vi "writeToXML.vi"(8 "error in (no error)":errorcluster, 10 "classLabel":string, 11 "SetEngineerAccessMode in":refnum<class "SetEngineerAccessMode.lvclass">) -> (0 "error out":errorcluster, 2 "XML out":string, 3 "SetEngineerAccessMode out":refnum<class "SetEngineerAccessMode.lvclass">)   [LabVIEW 2022 SP3, in "TCSDataDefinitions.lvlib" / "TCSCommand.lvlib" / "SetAccessMode.lvlib" / "SetEngineerAccessMode.lvclass"]
uses:
  SetEngineerAccessMode.lvclass
  SetEngineerAccessMode.lvclass/SetEngineerAccessMode.ctl
  SetAccessMode/SetAccessMode.lvclass
  <userlib>/Common/XML/XMLGenerator/XMLGenerator.lvclass
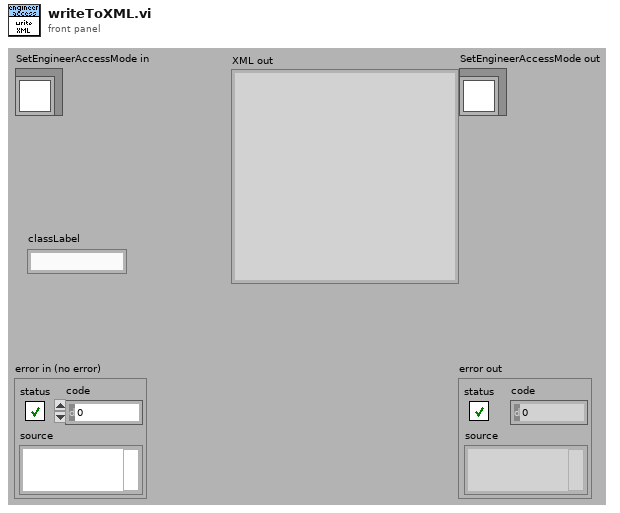
[diagram p1: front panel]
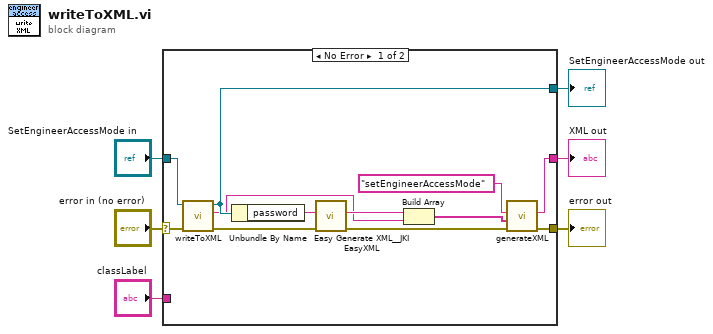
[diagram p0: block diagram]
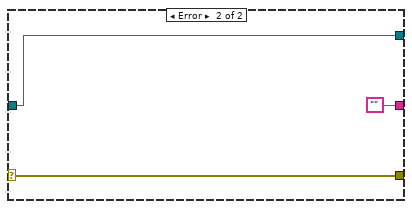
[diagram p2: hidden frame]
diagram:
  n1 = case shown="No Error" "error in (no error)" {
    selector: "error in (no error)" -> [w9 w21]
    tunnel: [w8 w21] -> w5
    tunnel: [w17 w20] -> w3
    tunnel: "SetEngineerAccessMode in" -> [w18 w20]
    tunnel: [w7 ""] -> w2
    tunnel: "classLabel" -> [_ _]
    frame No Error {
      n2 = call-parent "writeToXML.vi"("error in (no error)"=w9, "SetAccessMode in"=w18) -> ("error out"=w11:errorcluster, "XML out"=w14:string, "SetAccessMode out"=w17:refnum<class "SetEngineerAccessMode.lvclass">)  [unwired: 7 in]
      n3 = Unbundle By Name(w17) -> ("password"=w16:string)
      n4 = call <vilib>:"Easy Generate XML__JKI EasyXML.vi"("error in (no error)"=w11, "LabVIEW Data"=w16) -> ("error out"=w10:errorcluster, "XML String"=w15:string)  [unwired: 8 in]
      n5 = Build Array(w15, w14) -> (w13:string[])
      n6 = call <userlib>:"generateXML.vi"("error in"=w10, "childrenXML"=w13, "elementName"="setEngineerAccessMode" ("Class Label")) -> ("error out"=w8:errorcluster, "XML out"=w7:string)  [unwired: 6 in, 1 out]
    }
    frame Error {
    }
  }
  "error out" <- w5
  "SetEngineerAccessMode out" <- w3
  "XML out" <- w2
